vi "Initialize Matrix.vi"(6 "Control Ref Cluster":T1, 8 "error in (no error)":errorcluster, 11 "Main Frame Color":u32(colorbox)) -> (0 "error out":errorcluster)   [LabVIEW 2017, in "XY Plot Matrix.lvclass"]
uses:
  <vilib>/Math Plots/2D Math Plots/XY Plot Matrix/XY Plot Matrix/XY Plot Matrix.lvclass
  <vilib>/Math Plots/2D Math Plots/2D Plot/Action String/XYPlotMatrix Ctrl Act Cluster.ctl
  <vilib>/Math Plots/2D Math Plots/2D Plot/Action String/2DMathPlot State Class.ctl
  <vilib>/Math Plots/Plot Private Lib/NI_Math Plot Private Lib.lvlib
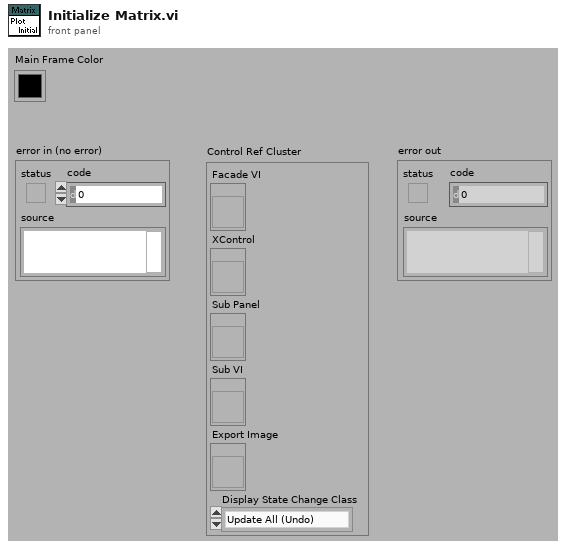
[diagram p1: front panel]
types:
  T1 = typedef "XYPlotMatrix Ctrl Act Cluster.ctl" = cluster{"Facade VI":refnum<vi>, "XControl":refnum<vi>, "Sub Panel":refnum<vi>, "Sub VI":refnum<vi>, "Export Image":refnum<vi>, "Display State Change Class":T2}
  T2 = typedef "2DMathPlot State Class.ctl" = enum16{"Update All (Undo)", "Update General", "Update Appearance", "Update Format", "Update Scale", "Update Marker", "Update Cursor", "None"}
  T3 = enum16{"No Scaling", "Scale All Objects", "Scale Single Object"}
  T4 = enum16{"Always On", "Always Off", "Off While Running"}
  T5 = typedef "LVBoundsTypeDef.ctl" = cluster{"Width":u32, "Height":u32}
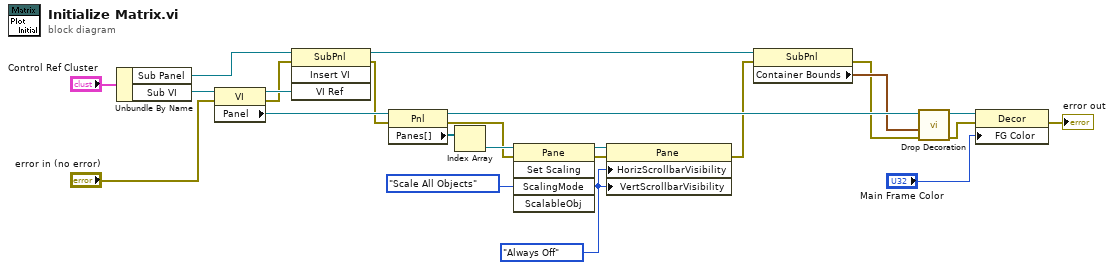
[diagram p0: block diagram]
diagram:
  w21 = T4."Always Off" ("Horizontal Scrollbar Visibility")
  n1 = Unbundle By Name("Control Ref Cluster") -> ("Sub Panel"=w18:refnum<vi>, "Sub VI"=w23:refnum<vi>)
  n2 = property class="VI"(reference=w23, error in="error in (no error)") -> (reference out=w17:refnum<vi>, error out=w9:errorcluster, "Panel"=w16:refnum<vi>)
  n3 = invoke class="SubPnl" method="Insert VI"(reference=w18, error in=w9, "VI Ref"=w17) -> (reference out=w8:refnum<vi>, error out=w10:errorcluster)  [unwired: 1 in, 2 out]
  n4 = property class="Pnl"(reference=w16, error in=w10) -> (reference out=w19:refnum<vi>, error out=w12:errorcluster, "Panes[]"=w20:refnum<vi>[])
  n5 = Index Array(array=w20) -> (element=w14:refnum<vi>)  [unwired: 1 in]
  n6 = invoke class="Pane" method="Set Scaling"(reference=w14, error in=w12, "ScalingMode"=T3."Scale All Objects" ("Scaling Mode")) -> (reference out=w13:refnum<vi>, error out=w11:errorcluster)  [unwired: 2 in, 3 out]
  n7 = property class="Pane"(reference=w13, error in=w11, "HorizScrollbarVisibility"=w21, "VertScrollbarVisibility"=w21) -> (error out=w6:errorcluster)  [unwired: 1 out]
  n8 = property class="SubPnl"(reference=w8, error in=w6) -> (error out=w5:errorcluster, "Container Bounds"=w7:T5)  [unwired: 1 out]
  n9 = call <vilib>:"Drop Decoration.vi"("error in (no error)"=w5, "Container Bounds"=w7, "Panel"=w19) -> ("error out"=w2:errorcluster, "Decoration refnum"=w4:refnum<vi>)  [unwired: 7 out]
  n10 = property class="Decor"(reference=w4, error in=w2, "FG Color"="Main Frame Color") -> (error out=→"error out":errorcluster)  [unwired: 1 out]
